vi "CloseDMM.vi"(8 "error in (no error)":errorcluster, 11 "DMM":refnum<visa-resource-name>="COM1") -> (0 "error out":errorcluster)   [LabVIEW 2015]
uses:
  <instrlib>/BK Precision 178XB Series/BK Precision 178XB Series.lvlib
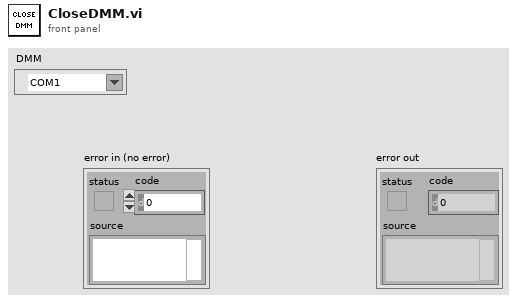
[diagram p1: front panel]
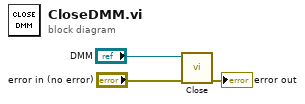
[diagram p0: block diagram]
diagram:
  n1 = call <instrlib>:"Close.vi"("error in (no error)"="error in (no error)", "VISA resource name"="DMM") -> ("error out"=→"error out":errorcluster)  [unwired: 9 in]
